vi "Main.vi"() -> ()   [LabVIEW 2015]
uses:
  TypeDefs/Queue Data.ctl
  SubVIs/App Data.vi
  SubVIs/App Strings.vi
  FGV/Timer Actions.ctl
  Desktop/Global 4.vi
panel:
  in  "Device name 2":tag="myDAQ1"
  in  "Time [ms] 2":dbl
  in  "Frequency 2":dbl
  in  "Period [s]":dbl
  in  "Device name":tag="myDAQ1"
  out "Time Elapsed":dbl format="%<%M:%S>t"
  out "Status":string
  in  "Time [ms]":dbl
  in  "Frequency":dbl
  in  "Stop Button":bool
  in  "Acquire Button":bool
  out "Waveform Graph":dbl[](graph)
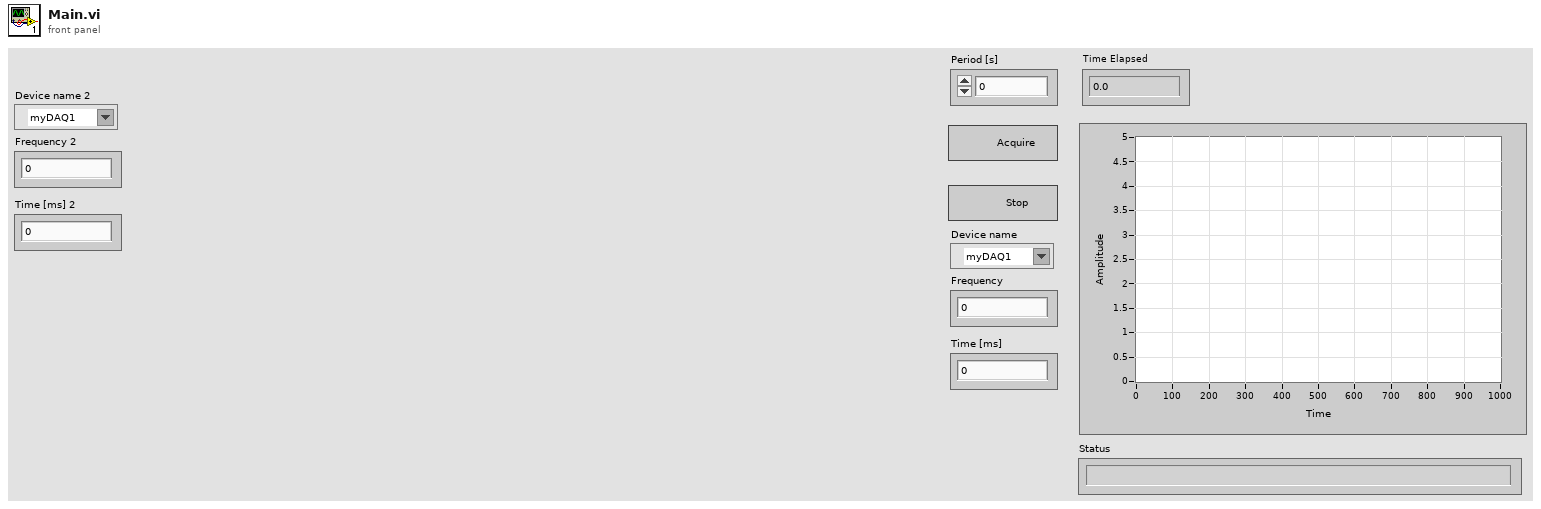
[diagram p1: front panel]
types:
  T1 = typedef "Timer Actions.ctl" = enum16{"Reset", "Get"}
  T2 = typedef "Queue Data.ctl" = cluster{"Action":string}
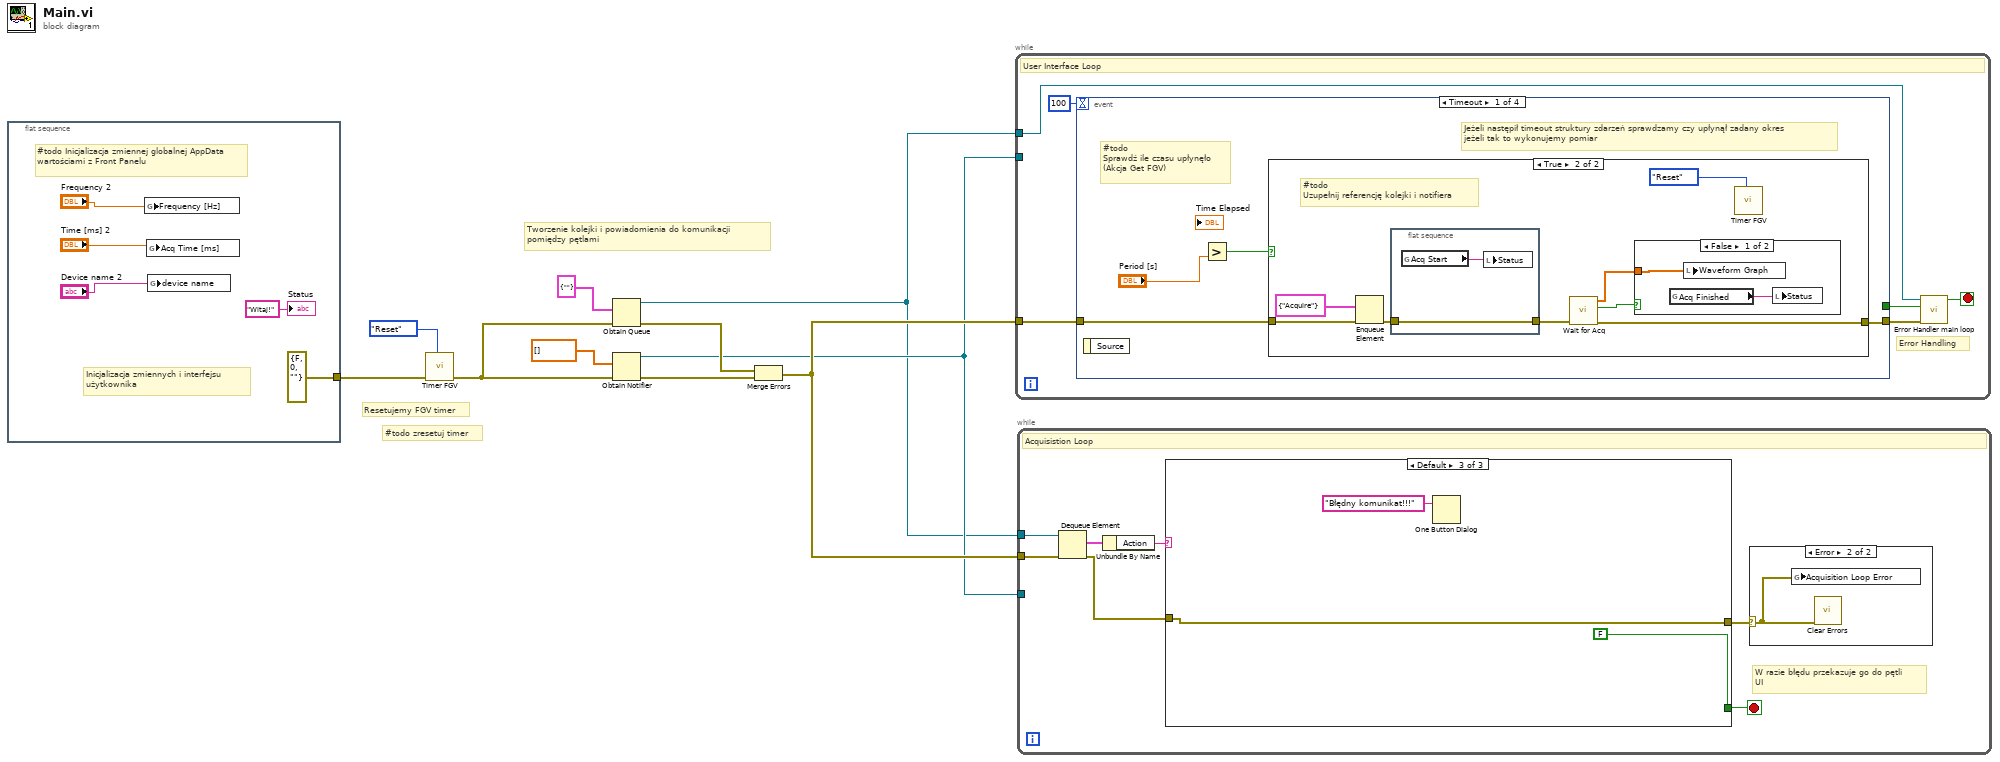
[diagram p0: block diagram]
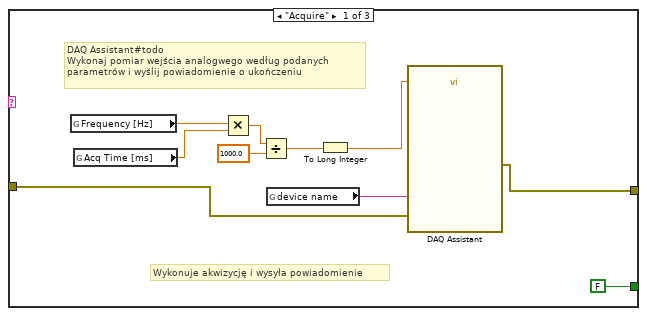
[diagram p3: hidden frame]
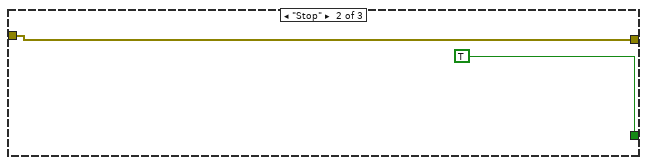
[diagram p4: hidden frame]
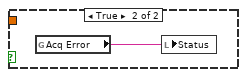
[diagram p6: hidden frame]
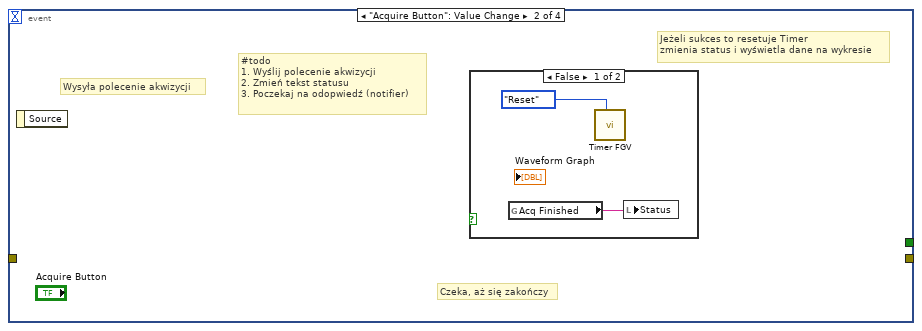
[diagram p7: hidden frame]
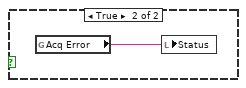
[diagram p8: hidden frame]
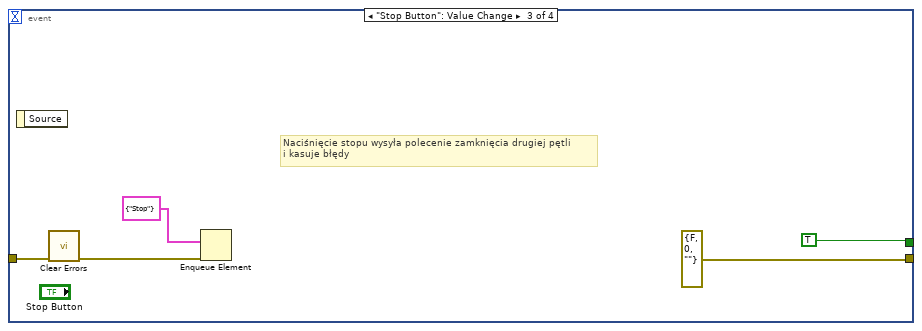
[diagram p9: hidden frame]
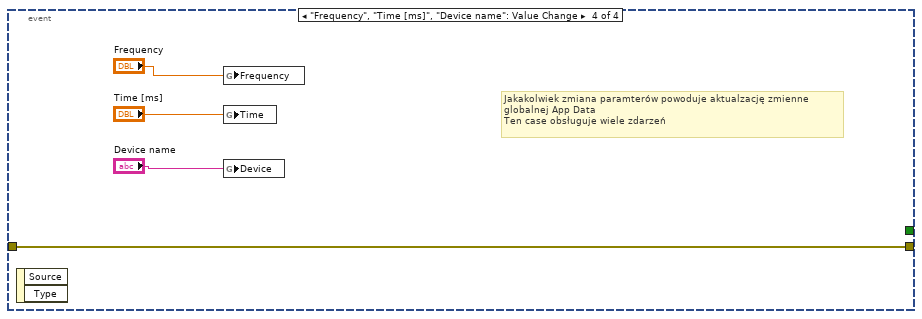
[diagram p10: hidden frame]
diagram:
  # "#todo zresetuj timer"
  # "Resetujemy FGV timer"
  # "Tworzenie kolejki i powiadomienia do komunikacji \npomiędzy pętlami"
  n1 = flat-sequence {
    tunnel: [errorcluster {"status"=FALSE, "code"=0, "source"=""} ("error constant")] -> w3
    frame #0 {
      # "#todo Inicjalizacja zmiennej globalnej AppData wartościami z Front Panelu"
      # "Inicjalizacja zmiennych i interfejsu \nużytkownika"
      n2 = global write "App Data.vi" "Frequency [Hz]"("Frequency 2") -> ()
      n3 = global write "App Data.vi" "Acq Time [ms]"("Time [ms] 2") -> ()
      n4 = global write "App Data.vi" "device name"("Device name 2") -> ()
      "Status" <- "Witaj!" ("Status")
    }
  }
  n5 = call "Timer FGV.vi"("Action"=Timer_Actions."Reset", "error in (no error)"=w3) -> ("error out"=w2:errorcluster)  [unwired: 8 in, 1 out]
  n6 = Obtain Queue(element data type=T2 {"Action"=""}, error in (no error)=w2) -> (queue out=w4:refnum<queue>, error out=w9:errorcluster)  [unwired: 3 in, 1 out]
  n7 = Obtain Notifier(notification data type=dbl[] [], error in (no error)=w2) -> (notifier out=w5:refnum<notifier>, error out=w7:errorcluster)  [unwired: 2 in, 1 out]
  n8 = Merge Errors(w9, w7) -> (w6:errorcluster)
  n9 = while {
    tunnel: w6 -> [w20]
    tunnel: w4 -> [w16]
    tunnel: w5 -> [_]
    stop <- w17 stop-if-true
    # "Error Handling"
    # "User Interface Loop"
    n10 = event shown="[0] Timeout" {
      selector: _ -> [_ _ _ _]
      dyn-events: _ -> [_ _ _ _]
      timeout: 100 -> [_ _ _ _]
      tunnel: w20 -> [w23 _ w44 w51]
      tunnel: [w22 _ errorcluster {"status"=FALSE, "code"=0, "source"=""} ("error constant") w51] -> w18
      tunnel: [_ _ TRUE _] -> w19
      event Timeout {
        # "#todo\nSprawdź ile czasu upłynęło\n(Akcja Get FGV)"
        # "Jeżeli następił timeout struktury zdarzeń sprawdzamy czy upłynął zadany okres \njeżeli tak to wykonujemy pomiar"
        n11 = event-data() -> ()  [unwired: 1 in, 1 out]
        n12 = Greater?(y="Period [s]") -> (0:w24:bool)  [unwired: 1 in]
        n13 = case shown="True" w24 {
          tunnel: w23 -> [w26 w34]
          tunnel: [w26 w27] -> w22
          frame False {
          }
          frame True {
            # "#todo\nUzupełnij referencję kolejki i notifiera"
            n14 = Enqueue Element(element=T2 {"Action"="Acquire"}, error in (no error)=w34) -> (error out=w32:errorcluster)  [unwired: 2 in, 2 out]
            n15 = flat-sequence {
              tunnel: w32 -> [w38]
              tunnel: [w38] -> w31
              frame #0 {
                n16 = global read "App Strings.vi" "Acq Start"() -> (w39:string)
                n17 = local write "Status"(w39) -> ()
              }
            }
            n18 = call "Wait for Acq.vi"("error in (no error)"=w31) -> ("error out"=w27:errorcluster, "timed out?"=w28:bool, "Array"=w30:dbl[])  [unwired: 8 in]
            n19 = case shown="False" w28 {
              tunnel: w30 -> [w35 _]
              frame False {
                n20 = global read "App Strings.vi" "Acq Finished"() -> (w36:string)
                n21 = local write "Waveform Graph"(w35) -> ()
                n22 = local write "Status"(w36) -> ()
              }
              frame True {
                n23 = global read "App Strings.vi" "Acq Error"() -> (w37:string)
                n24 = local write "Status"(w37) -> ()
              }
            }
            n25 = call "Timer FGV.vi"("Action"=Timer_Actions."Reset") -> ()  [unwired: 9 in, 2 out]
          }
        }
      }
      event "Acquire Button": Value Change {
        # "#todo\n1. Wyślij polecenie akwizycji\n2. Zmień tekst statusu\n3. Poczekaj na odopwiedź (notifier)"
        # "Jeżeli sukces to resetuje Timer\nzmienia status i wyświetla dane na wykresie"
        # "Czeka, aż się zakończy"
        # "Wysyła polecenie akwizycji"
        n26 = event-data() -> ()  [unwired: 1 in, 1 out]
        n27 = case shown="False" {
          selector: _ -> [_ _]
          frame False {
            n28 = global read "App Strings.vi" "Acq Finished"() -> (w41:string)
            n29 = call "Timer FGV.vi"("Action"=Timer_Actions."Reset") -> ()  [unwired: 9 in, 2 out]
            n30 = local write "Status"(w41) -> ()
          }
          frame True {
            n31 = global read "App Strings.vi" "Acq Error"() -> (w42:string)
            n32 = local write "Status"(w42) -> ()
          }
        }
      }
      event "Stop Button": Value Change {
        # "Naciśnięcie stopu wysyła polecenie zamknięcia drugiej pętli\ni kasuje błędy"
        n33 = event-data() -> ()  [unwired: 1 in, 1 out]
        n34 = call <vilib>:"Clear Errors.vi"("error in (no error)"=w44) -> ("error out"=w43:errorcluster)  [unwired: 5 in, 1 out]
        n35 = Enqueue Element(element=T2 {"Action"="Stop"}, error in (no error)=w43) -> ()  [unwired: 2 in, 3 out]
      }
      event "Frequency", "Time [ms]", "Device name": Value Change {
        # "Jakakolwiek zmiana paramterów powoduje aktualzację zmienne \nglobalnej App Data\nTen case obsługuje wiele zdarzeń"
        n36 = event-data() -> ()  [unwired: 1 in, 2 out]
        n37 = global write "Global 4.vi" "Frequency"("Frequency") -> ()
        n38 = global write "Global 4.vi" "Time"("Time [ms]") -> ()
        n39 = global write "Global 4.vi" "Device"("Device name") -> ()
      }
    }
    n40 = call "Error Handler main loop.vi"("error in (no error)"=w18, "Exit?"=w19, "Queue in"=w16) -> ("Exit?"=w17:bool)  [unwired: 8 in]
  }
  n41 = while {
    tunnel: w6 -> [w56]
    tunnel: w4 -> [w55]
    tunnel: w5 -> [_]
    stop <- w53 stop-if-true
    # "W razie błędu przekazuje go do pętli\nUI"
    # "Acquisistion Loop"
    n42 = Dequeue Element(queue=w55, error in (no error)=w56) -> (element=w58:T2, error out=w54:errorcluster)  [unwired: 1 in, 2 out]
    n43 = Unbundle By Name(w58) -> ("Action"=w57:string)
    n44 = case shown="Default" w57 {
      tunnel: w54 -> [w61 w69 w72]
      tunnel: [FALSE TRUE FALSE] -> w53
      tunnel: [w60 w69 w72] -> w52
      frame "Acquire" {
        # "DAQ Assistant#todo\nWykonaj pomiar wejścia analogwego według podanych \nparametrów i wyślij powiadomienie o ukończeniu"
        # "Wykonuje akwizycję i wysyła powiadomienie"
        n45 = global read "App Data.vi" "Frequency [Hz]"() -> (w66:dbl)
        n46 = global read "App Data.vi" "Acq Time [ms]"() -> (w65:dbl)
        n47 = Multiply(x=w66, y=w65) -> (x*y=w63:dbl)
        n48 = Divide(x=w63, y=1000.0) -> (x/y=w62:dbl)
        n49 = global read "App Data.vi" "device name"() -> (w67:tag)
        n50 = To Long Integer() -> ()  [unwired: 1 in, 1 out]
        n51 = call "DAQ Assistant"("number of samples"=w62, "error in"=w61, "device name"=w67) -> ("error out"=w60:errorcluster)  [unwired: 14 in, 2 out]
      }
      frame "Stop" {
      }
      frame Default {
        n52 = One Button Dialog(message="Błędny komunikat!!!") -> ()  [unwired: 1 in, 1 out]
      }
    }
    n53 = case shown="Error" w52 {
      selector: w52 -> [_ w59]
      frame No Error {
      }
      frame Error {
        n54 = global write "App Data.vi" "Acquisition Loop Error"(w59) -> ()
        n55 = call <vilib>:"Clear Errors.vi"("error in (no error)"=w59) -> ()  [unwired: 5 in, 2 out]
      }
    }
  }
